vi "GetText.vi"(8 "error in":errorcluster, 11 "EngineTags in":refnum<class "Engine Mappings.lvclass">) -> (0 "error out":errorcluster, 1 "additional text":string, 2 "text":string, 3 "EngineTags out":refnum<class "Engine Mappings.lvclass">, 4 "glyph":string)   [LabVIEW 2013, in "PL Framework Configuration Tool.lvlib" / "Engine Mappings.lvclass"]
uses:
  Engine Mappings.lvclass
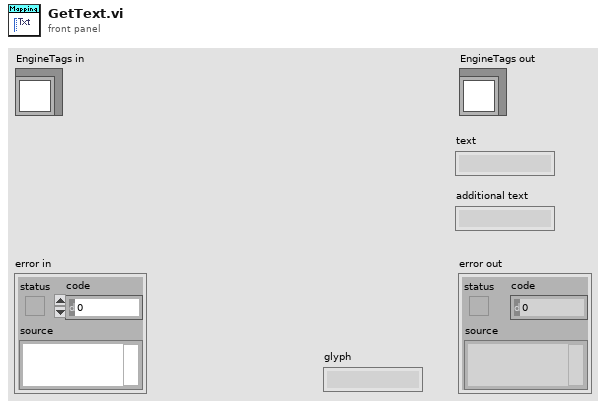
[diagram p1: front panel]
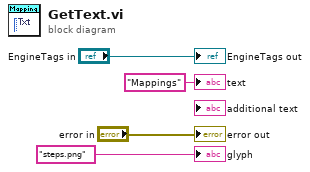
[diagram p0: block diagram]
diagram:
  "error out" <- "error in"
  "EngineTags out" <- "EngineTags in"
  "text" <- "Mappings" ("text")
  "glyph" <- "steps.png" ("glyph")
